vi "MW_Display_Py_Stop_Capture.vi"(0 "session in":refnum<k35>, 5 "module path":path=path "D:/dev/Guy_Storage/Work/Cancun/MW_Display_Test/Magewell Capture/Capture_LV.py", 11 "error in":errorcluster) -> (4 "session out":refnum<k35>, 6 "module path out":path, 14 "Stop Capture Success":bool, 15 "error out":errorcluster)   [LabVIEW 2023]
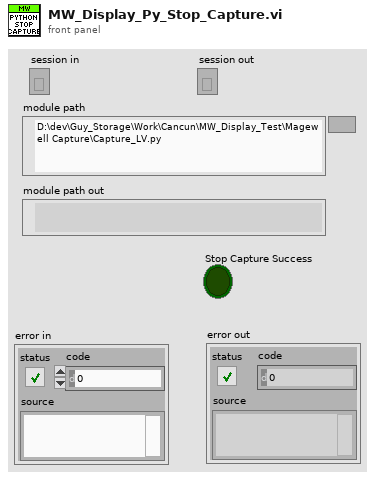
[diagram p1: front panel]
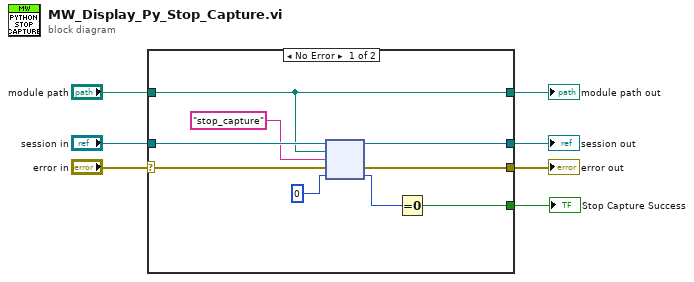
[diagram p0: block diagram]
diagram:
  n1 = case shown="No Error" "error in" {
    selector: "error in" -> [w13 w18]
    tunnel: "module path" -> [w11 w17]
    tunnel: "session in" -> [w16 w19]
    tunnel: [w15 w18] -> w3
    tunnel: [w14 w19] -> w5
    tunnel: [w11 w17] -> w2
    tunnel: [w8 _] -> w1
    frame No Error {
      n2 = node(w16, w11, "stop_capture" ("function name"), w13, 0) -> (w14:refnum<k35>, w15:errorcluster, w9:i32)  [unwired: 2 out]
      n3 = Equal To 0?(x=w9) -> (x = 0?=w8:bool)
    }
    frame Error {
    }
  }
  "session out" <- w5
  "error out" <- w3
  "module path out" <- w2
  "Stop Capture Success" <- w1
